vi "TEST Delete Duplicate Key.vi"() -> ()   [LabVIEW 2013, in "Carya Config.lvclass"]
doc: "Copyright 2018, Carya Automatisering, Wiebe Walstra."
uses:
  Carya Config.lvclass
  Carya Config (By Reference)/Carya Config (By Reference).lvclass
panel:
  out "String 3":string
  out "String 2":string
  out "String":string
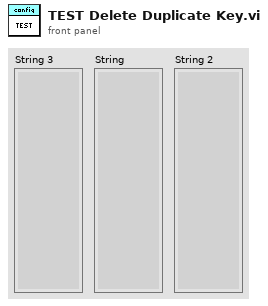
[diagram p1: front panel]
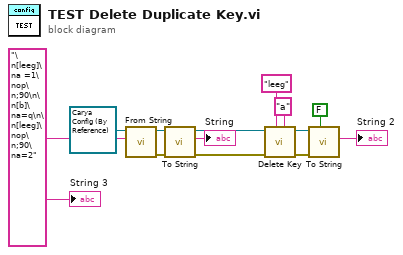
[diagram p0: block diagram]
diagram:
  w8 = "\n[leeg]\na =1\nop\n;90\n\n[b]\na=q\n\n[leeg]\nop\n;90\na=2" ("String")
  n1 = call-dynamic "From String.vi"("String"=w8, "Carya Config in"=refnum<class "Carya Config (By Reference).lvclass"> refnum) -> ("error out"=w11:errorcluster, "Carya Config out"=w13:refnum<class "Carya Config (By Reference).lvclass">)  [unwired: 7 in, 1 out]
  n2 = call-dynamic "To String.vi"("error in (no error)"=w11, "Carya Config in"=w13) -> ("error out"=w4:errorcluster, "String"=→"String":string, "Carya Config out"=w5:refnum<class "Carya Config (By Reference).lvclass">)  [unwired: 7 in]
  n3 = call-dynamic "Delete Key.vi"("Key name"="a", "Section name"="leeg", "error in (no error)"=w4, "Carya Config in"=w5) -> ("error out"=w1:errorcluster, "Carya Config out"=w10:refnum<class "Carya Config (By Reference).lvclass">)  [unwired: 4 in, 2 out]
  n4 = call-dynamic "To String.vi"("Persitant only? [T]"=FALSE ("Persitant only?"), "error in (no error)"=w1, "Carya Config in"=w10) -> ("String"=→"String 2":string)  [unwired: 6 in, 2 out]
  "String 3" <- w8
